vi "AutoForceStore.vi"(11 "Command Cluster":T1) -> ()   [LabVIEW 2015]
uses:
  Common Code/commandCluster.ctl
  Robot Global Data.vi
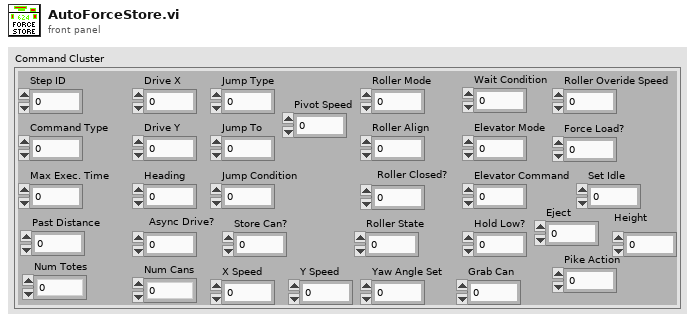
[diagram p1: front panel]
types:
  T1 = typedef "commandCluster.ctl" = cluster{"Step ID":i16, "Command Type":i16, "Drive X":sgl, "Drive Y":sgl, "Heading":sgl, "Max Exec. Time":i16, "Jump Type":i32, "Jump To":i16, "Jump Condition":i16, "Async Drive?":i16, "Roller Mode":i16, "Roller Align":i16, "Roller Closed?":i16, "Wait Condition":i16, "Elevator Mode":i16, "Elevator Command":i16, "Roller State":i16, "Hold Low?":i16, "Num Totes":i16, "Num Cans":dbl, "Past Distance":dbl, "Store Can?":dbl, "X Speed":dbl, "Y Speed":dbl, "Yaw Angle Set":dbl, "Grab Can":dbl, "Roller Overide Speed":dbl, "Force Load?":sgl, "Set Idle":sgl, "Eject":sgl, "Pike Action":sgl, "Pivot Speed":dbl, "Height":dbl}
  T2 = typedef "Elevator Control Command.ctl" = cluster{"Command":T3, "Manual Motor Out":dbl, "Manual Eject Piston":bool, "Mode":T4, "Override Limits":bool, "Manual Stabilizer":bool, "Manual Finger":bool, "Store Trashcan?":bool, "Hold Low?":bool, "Idle Mode":T5, "HP Load":bool, "Unstick":bool, "Raw Height Set":dbl, "Force Store":bool}
  T3 = typedef "Elevator Command.ctl" = enum16{"Idle", "Load 1", "Load 2", "Load 3", "Drop Stack", "Eject Stack", "Untip Trashcan", "Load Trashcan", "HP Load", "HP Score"}
  T4 = typedef "Elevator Mode.ctl" = enum16{"Manual", "Safe", "Auto"}
  T5 = typedef "Elevator Idle Mode.ctl" = enum16{"Load 1", "Load 2", "Load 3", "Load Can", "Untip Can", "Step Load", "Drop Stack", "Raw Height"}
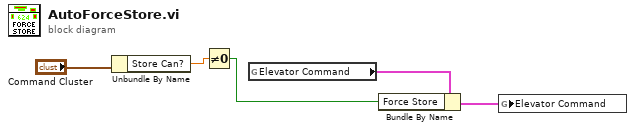
[diagram p0: block diagram]
diagram:
  n1 = Unbundle By Name("Command Cluster") -> ("Store Can?"=w5:dbl)
  n2 = Not Equal To 0?(x=w5) -> (x != 0?=w1:bool)
  n3 = global read "Robot Global Data.vi" "Elevator Command"() -> (w3:T2)
  n4 = Bundle By Name(cluster=w3, "Force Store"=w1) -> (w2:T2)
  n5 = global write "Robot Global Data.vi" "Elevator Command"(w2) -> ()
